vi "3.3.vi"() -> ()   [LabVIEW 2020]
panel:
  out "r^2":dbl[](array[numeric])
  out "r":dbl[](array[numeric])
  out "XY Graph":cluster{dbl[], dbl[]}(graph)
  in  "B":dbl
  in  "A":dbl
  out "Array":dbl[](array[numeric])
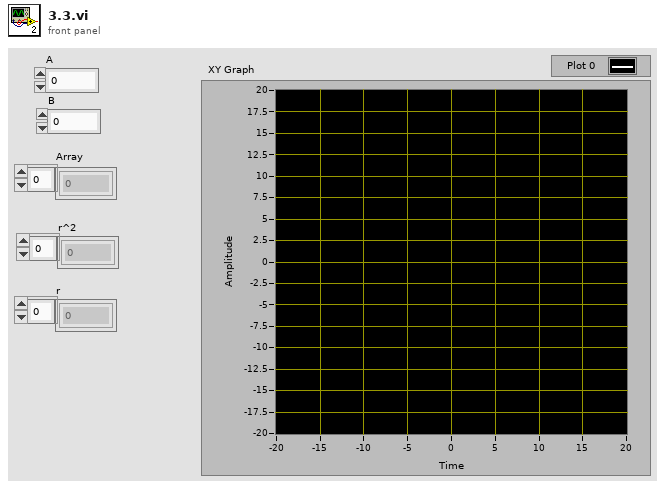
[diagram p1: front panel]
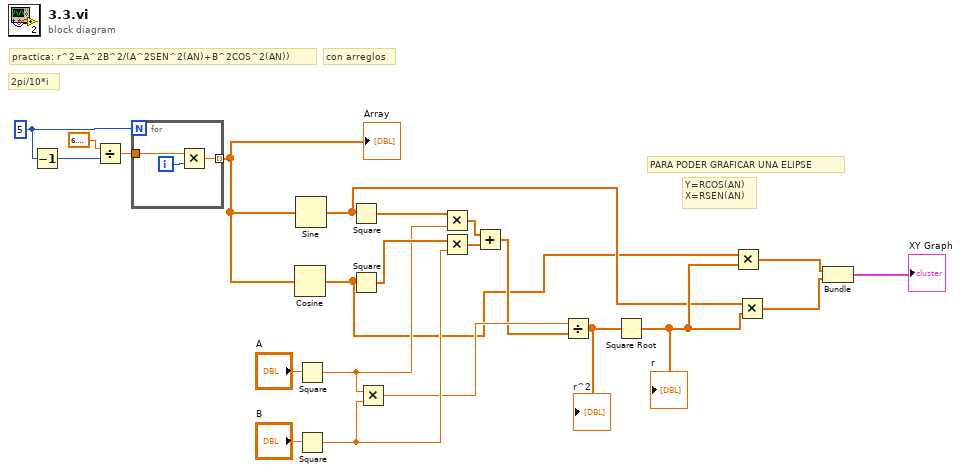
[diagram p0: block diagram]
diagram:
  w21 = 5
  # "PARA PODER GRAFICAR UNA ELIPSE"
  # "Y=RCOS(AN)\nX=RSEN(AN)"
  # "con arreglos"
  # "2pi/10*i"
  # "practica: r^2=A^2B^2/(A^2SEN^2(AN)+B^2COS^2(AN))"
  n1 = Decrement(x=w21) -> (x-1=w20:i32)
  n2 = Divide(x=6.283185307179586, y=w20) -> (x/y=w19:dbl)
  n3 = for {
    N: w21 -> [_]
    tunnel: w19 -> [w25]
    tunnel: [w23] -> w18 mode=indexing
    i -> [w24]
    n4 = Multiply(x=w25, y=w24) -> (x*y=w23:dbl)
  }
  "Array" <- w18
  n5 = Cosine(x=w18) -> (cos(x)=w4:dbl[])
  n6 = Sine(x=w18) -> (sin(x)=w5:dbl[])
  n7 = Square(x="A") -> (x^2=w13:dbl)
  n8 = Square(x="B") -> (x^2=w12:dbl)
  n9 = Square(x=w5) -> (x^2=w15:dbl[])
  n10 = Square(x=w4) -> (x^2=w14:dbl[])
  n11 = Multiply(x=w13, y=w12) -> (x*y=w9:dbl)
  n12 = Multiply(x=w15, y=w13) -> (x*y=w11:dbl[])
  n13 = Multiply(x=w14, y=w12) -> (x*y=w10:dbl[])
  n14 = Add(x=w11, y=w10) -> (x+y=w8:dbl[])
  n15 = Divide(x=w9, y=w8) -> (x/y=w7:dbl[])
  "r^2" <- w7
  n16 = Square Root(x=w7) -> (sqrt(x)=w6:dbl[])
  "r" <- w6
  n17 = Multiply(x=w4, y=w6) -> (x*y=w3:dbl[])
  n18 = Multiply(x=w5, y=w6) -> (x*y=w2:dbl[])
  n19 = Bundle(w3, w2) -> (→"XY Graph":cluster{dbl[], dbl[]})  [unwired: 1 in]
